vi "get_total_number_of_pixels_per_cycle.vi"(8 "error in (no error)":errorcluster, 11 "TrajectoryDL090201FrameScan in":refnum<class "TrajectoryDL090201FrameScan.lvclass">) -> (0 "error out":errorcluster, 2 "total number of pixels per cycle":i32, 3 "TrajectoryDL090201FrameScan out":refnum<class "TrajectoryDL090201FrameScan.lvclass">)   [LabVIEW 2010, in "TrajectoryDL090201FrameScan.lvclass"]
uses:
  TrajectoryDL090201FrameScan.lvclass
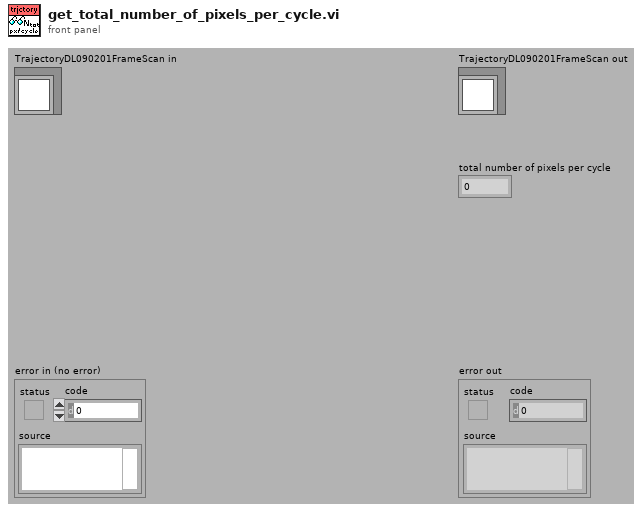
[diagram p1: front panel]
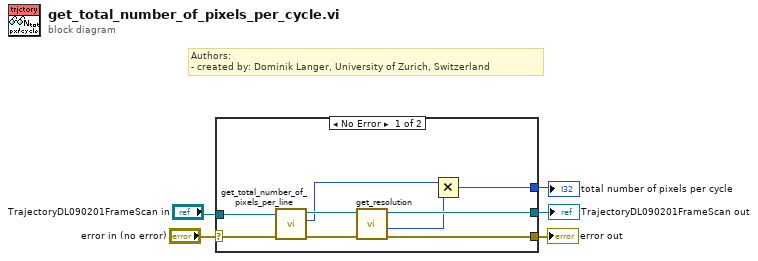
[diagram p0: block diagram]
diagram:
  # "Authors: \n- created by: Dominik Langer, University of Zurich, Switzerland"
  n1 = case shown="No Error" "error in (no error)" {
    selector: "error in (no error)" -> [w14 w16]
    tunnel: [w12 w16] -> w4
    tunnel: [w9 w15] -> w2
    tunnel: "TrajectoryDL090201FrameScan in" -> [w10 w15]
    tunnel: [w6 _] -> w1
    frame No Error {
      n2 = call-dynamic "get_total_number_of_pixels_per_line.vi"("error in (no error)"=w14, "DL090201FrameScanTrajectory in"=w10) -> ("error out"=w13:errorcluster, "total number of pixels per line"=w7:i32, "DL090201FrameScanTrajectory out"=w11:refnum<class "TrajectoryDL090201FrameScan.lvclass">)  [unwired: 7 in]
      n3 = call-dynamic "get_resolution.vi"("error in (no error)"=w13, "TrajectoryDL090201FrameScan in"=w11) -> ("error out"=w12:errorcluster, "y"=w8:i32, "TrajectoryDL090201FrameScan out"=w9:refnum<class "TrajectoryDL090201FrameScan.lvclass">)  [unwired: 6 in, 1 out]
      n4 = Multiply(x=w7, y=w8) -> (x*y=w6:i32)
    }
    frame Error {
    }
  }
  "error out" <- w4
  "TrajectoryDL090201FrameScan out" <- w2
  "total number of pixels per cycle" <- w1
